vi "Mix Mono To Stereo.vi"(11 "Audio Data":waveform(i16)[](array[waveform])) -> (3 "Audio Data Out":waveform(i16)[](array[waveform]))   [LabVIEW 2019, in "Audio Processing.lvlib"]
doc: "Upmix a single channel wavform to a stereo waveform by duplicating the single channel into two channels."
uses:
  Audio Processing.lvlib
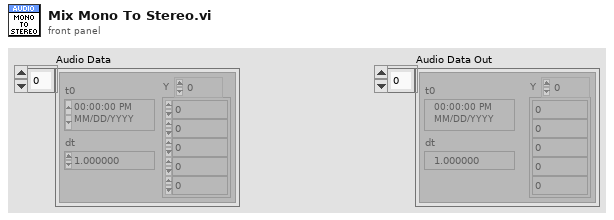
[diagram p1: front panel]
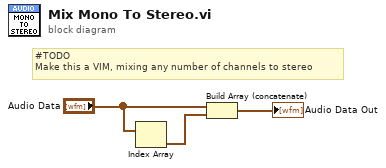
[diagram p0: block diagram]
diagram:
  # "#TODO\nMake this a VIM, mixing any number of channels to stereo"
  n1 = Index Array(array="Audio Data") -> (element=w2:waveform(i16))  [unwired: 1 in]
  n2 = Build Array (concatenate)("Audio Data", w2) -> (→"Audio Data Out":waveform(i16)[])
